vi "cuenta pulsos y duracion.vi"(11 "Array 2":dbl[](array[numeric])) -> (1 "flancos negativos":i32[](array[numeric]), 2 "flancos positivos":i32[](array[numeric]), 3 "size(s)":i32)   [LabVIEW 2021]
panel:
  out "Array":dbl[](array[numeric])
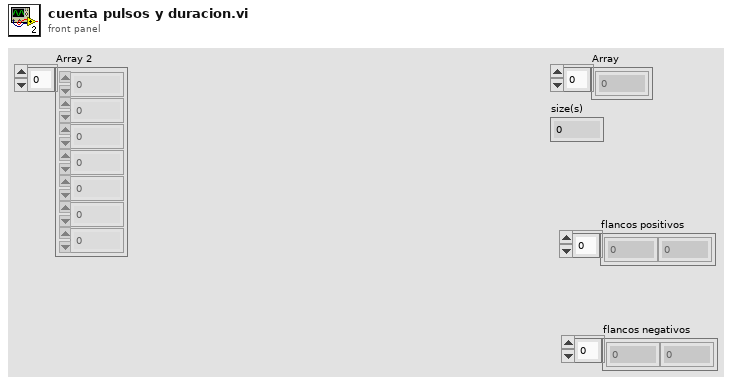
[diagram p1: front panel]
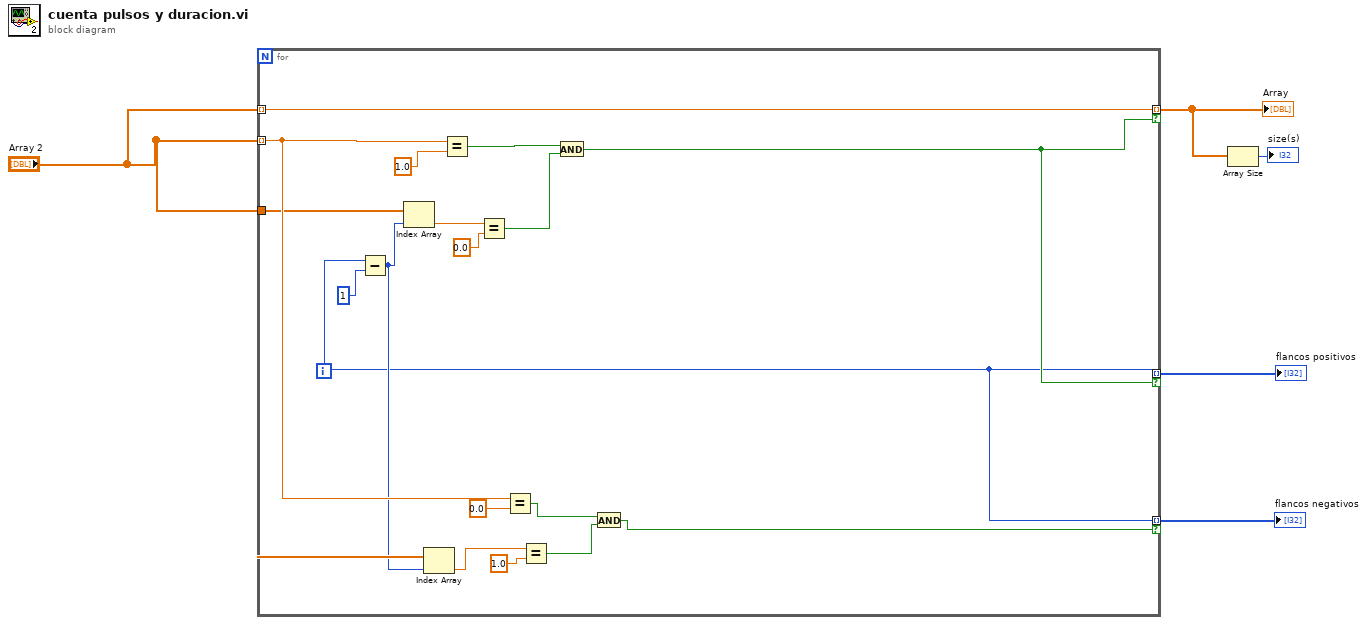
[diagram p0: block diagram]
diagram:
  n1 = for {
    tunnel: "Array 2" -> [w17] mode=indexing
    tunnel: "Array 2" -> [w15] mode=indexing
    tunnel: "Array 2" -> [w13]
    tunnel: [w17] -> w3 mode=indexing if=w16
    tunnel: [w7] -> w1 mode=indexing if=w16
    tunnel: [w7] -> w2 mode=indexing if=w6
    i -> [w7]
    n2 = Subtract(x=w7, y=1) -> (x-y=w12:i32)
    n3 = Index Array(array=w13, index=w12) -> (element=w21:dbl)
    n4 = Index Array(array=w13, index=w12) -> (element=w11:dbl)
    n5 = Equal?(x=w15, y=1.0) -> (x = y?=w18:bool)
    n6 = Equal?(x=w21, y=0.0) -> (x = y?=w19:bool)
    n7 = Equal?(x=w15, y=0.0) -> (x = y?=w9:bool)
    n8 = Equal?(x=w11, y=1.0) -> (x = y?=w8:bool)
    n9 = And(x=w18, y=w19) -> (x .and. y?=w16:bool)
    n10 = And(x=w9, y=w8) -> (x .and. y?=w6:bool)
  }
  "Array" <- w3
  "flancos positivos" <- w1
  "flancos negativos" <- w2
  n11 = Array Size(array=w3) -> (size(s)=→"size(s)":i32)
